vi "Begin.vi"(8 "error in":errorcluster) -> (0 "error out":errorcluster)   [LabVIEW 2017]
doc: "Called before other user functions, this VI is expected to open initial I/O refnums, load in file data, and do all program initialization. Notice that the <B>error out</B> terminal is simply used for data flow. Wiring it to other structures or subVIs ensures that this VI runs first."
uses:
  <vilib>/Rock Robotics/WPI/DriverStation/WPI_DriverStationRobotMode2.ctl
  <vilib>/Rock Robotics/WPI/Joystick/WPI_JoystickDeviceEnum.ctl
  <vilib>/Rock Robotics/WPI/Solenoid/WPI_SolenoidChannel.ctl
  <vilib>/Rock Robotics/SystemInterfaces/DIO/FPGA_DIOChannel.ctl
  Robot Global Data.vi
  <vilib>/Rock Robotics/WPI/Solenoid/WPI_SolenoidOpenSingle.vi
  <vilib>/Rock Robotics/WPI/Counter/WPI_CounterDigitalInputToDigitalSource.vi
  <vilib>/Rock Robotics/WPI/Switch/WPI_SwitchOpenLimit.vi
  <vilib>/Rock Robotics/WPI/Utilities/WPI_GetSetVariantRefNum.vi
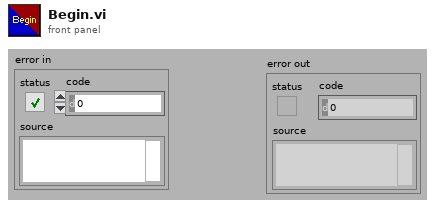
[diagram p1: front panel]
types:
  T1 = typedef "WPI_SolenoidChannel.ctl" = enum8{"Solenoid 0", "Solenoid 1", "Solenoid 2", "Solenoid 3", "Solenoid 4", "Solenoid 5", "Solenoid 6", "Solenoid 7", "Invalid"}
  T2 = typedef "FPGA_DIOChannel.ctl" = enum8{"DIO 0", "DIO 1", "DIO 2", "DIO 3", "DIO 4", "DIO 5", "DIO 6", "DIO 7", "DIO 8", "DIO 9", "DIO MXP 0", "DIO MXP 1", "DIO MXP 2", "DIO MXP 3", "DIO MXP 4", "DIO MXP 5", "DIO MXP 6", "DIO MXP 7", "DIO MXP 8", "DIO MXP 9", "DIO MXP 10", "DIO MXP 11", "DIO MXP 12", "DIO MXP 13", "DIO MXP 14", "DIO MXP 15", "SPI Port CS1", "SPI Port CS2", "SPI Port CS3", "SPI Port MISO", "SPI Port MOSI", "Invalid"}
  T3 = typedef "WPI_JoystickDeviceEnum.ctl" = enum16{"USB 0", "USB 1", "USB 2", "USB 3", "USB 4", "USB 5"}
  T4 = typedef "WPI_DriverStationRobotMode2.ctl" = enum16{"Autonomous Disabled", "Autonomous Enabled", "Teleop Disabled", "Teleop Enabled", "Disconnected", "Finish", "Test Disabled", "Test Enabled", "Emergency Stopped"}
  T5 = typedef "WPI_CompressorDevRef.ctl" = cluster{"DevStatus":errorcluster, "Pneumatics Control Module":u8}
  T6 = typedef "WPI_SwitchDevRef.ctl" = cluster{"DevStatus":errorcluster, "DIO Channel":T2, "CntIndex":T7, "Normally Closed":bool}
  T7 = typedef "FPGA_CounterCtrSystemIndex.ctl" = enum8{"Ctr 0", "Ctr 1", "Ctr 2", "Ctr 3", "Ctr 4", "Ctr 5", "Ctr 6", "Ctr 7", "Invalid"}
  T8 = typedef "WPI_DigitalInputDevRef.ctl" = cluster{"DevStatus":errorcluster, "DIO Channel":T2}
  T9 = typedef "WPI_SolenoidDevRef.ctl" = cluster{"DevStatus":errorcluster, "Pneumatics Control Module":u8, "Forward Solenoid Channel":T1, "Reverse Solenoid Channel":T1}
  T10 = typedef "FPGA_CounterEncoderSourceConvertionLVSourceType.ctl" = cluster{"DevStatus":errorcluster, "AnalogTriggerMode?":bool, "DigitalMode":cluster{"DIO Channel":T11}, "AnalogTriggerMode":cluster{"AnalogTriggerIndex":T12, "OutputType":T13}}
  T11 = typedef "FPGA_DIODigitalSourceChannel.ctl" = enum8{"DIO 0", "DIO 1", "DIO 2", "DIO 3", "DIO 4", "DIO 5", "DIO 6", "DIO 7", "DIO 8", "DIO 9", "DIO MXP 0", "DIO MXP 1", "DIO MXP 2", "DIO MXP 3", "DIO MXP 4", "DIO MXP 5", "DIO MXP 6", "DIO MXP 7", "DIO MXP 8", "DIO MXP 9", "DIO MXP 10", "DIO MXP 11", "DIO MXP 12", "DIO MXP 13", "DIO MXP 14", "DIO MXP 15", "Disabled"}
  T12 = typedef "FPGA_AnalogTriggerIndex.ctl" = enum8{"Trig 0", "Trig 1", "Trig 2", "Trig 3", "Trig 4", "Trig 5", "Trig 6", "Trig 7", "Invalid"}
  T13 = typedef "FPGA_AnalogTriggerOutType.ctl" = enum16{"InWindow", "TriggerState", "Rising", "Falling"}
  T14 = typedef "WPI_JoystickDevRef.ctl" = cluster{"Device":T3}
  T15 = typedef "WPI_EncoderDevRef.ctl" = cluster{"DevStatus":errorcluster, "EncoderIndex":T16, "CounterIndex":T7, "DistancePerCount":dbl, "Decoding Type":T17}
  T16 = typedef "FPGA_EncoderIdx.ctl" = enum8{"Enc 0", "Enc 1", "Enc 2", "Enc 3", "Enc 4", "Enc 5", "Enc 6", "Enc 7", "Invalid"}
  T17 = typedef "WPI_EncoderType.ctl" = enum16{"1x", "2x", "4x"}
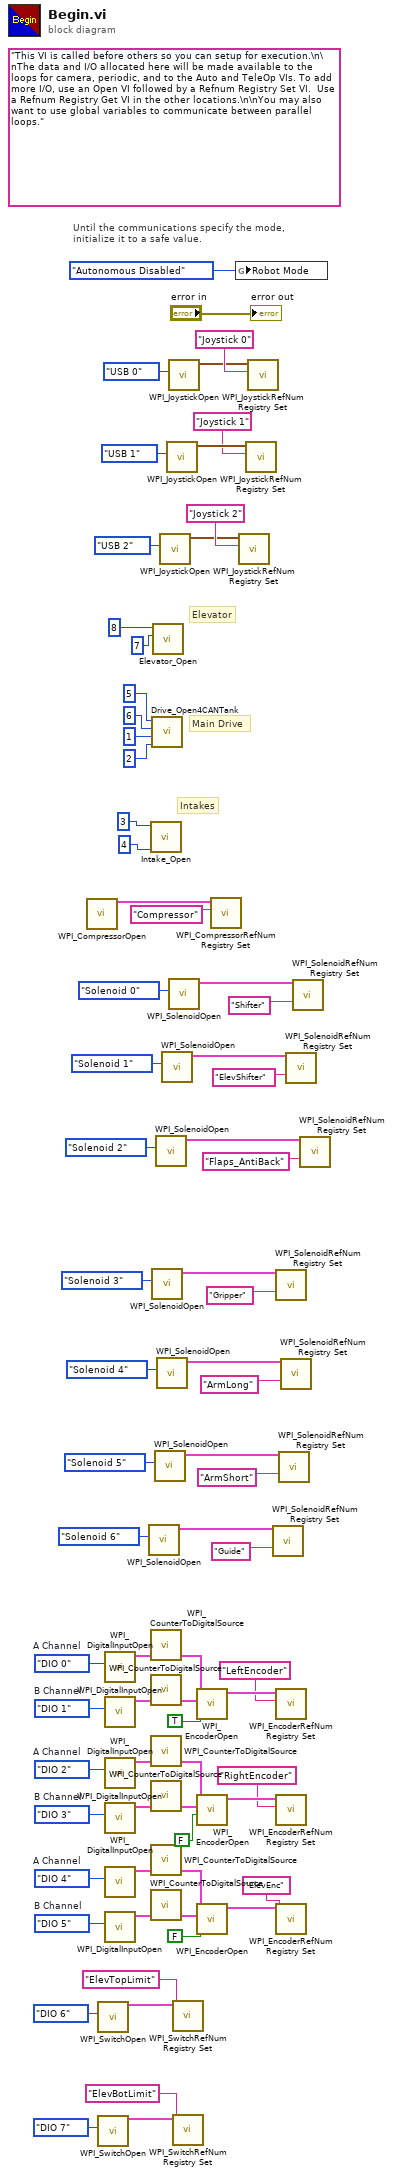
[diagram p0: block diagram]
diagram:
  w28 = FPGA_DIOChannel."DIO 5"  # B Channel
  w29 = FPGA_DIOChannel."DIO 4"  # A Channel
  w44 = FPGA_DIOChannel."DIO 3"  # B Channel
  w45 = FPGA_DIOChannel."DIO 2"  # A Channel
  w55 = FPGA_DIOChannel."DIO 1"  # B Channel
  w54 = FPGA_DIOChannel."DIO 0"  # A Channel
  (unwired) "This VI is called before others so you can setup for execution.\n\nThe data and I/O allocated here will be made available to the loops for camera, periodic, and to the Auto and TeleOp VIs. To add more I/O, use an Open VI followed by a Refnum Registry Set VI.  Use a Refnum Registry Get VI in the other locations.\n\nYou may also want to use global variables to communicate between parallel loops."
  # "Elevator"
  # "Intakes"
  # "Main Drive"
  # "Until the communications specify the mode,\ninitialize it to a safe value."
  n1 = call <vilib>:"WPI_CompressorOpen.vi"() -> ("CompressorDevRef"=w63:T5)  [unwired: 14 in, 1 out]
  n2 = call-poly <vilib>:"WPI_SwitchOpen.vi"("DIO Channel"=FPGA_DIOChannel."DIO 6") -> ("SwitchDevRef"=w15:T6)  [unwired: 9 in, 1 out]
  n3 = call-poly <vilib>:"WPI_SwitchOpen.vi"("DIO Channel"=FPGA_DIOChannel."DIO 7") -> ("SwitchDevRef"=w12:T6)  [unwired: 9 in, 1 out]
  n4 = call <vilib>:"WPI_DigitalInputOpen.vi"("DIO Channel"=w54) -> ("DigitalInputDevRef"=w51:T8)  [unwired: 1 in, 9 out]
  n5 = call <vilib>:"WPI_DigitalInputOpen.vi"("DIO Channel"=w55) -> ("DigitalInputDevRef"=w52:T8)  [unwired: 1 in, 9 out]
  n6 = call <vilib>:"WPI_DigitalInputOpen.vi"("DIO Channel"=w45) -> ("DigitalInputDevRef"=w48:T8)  [unwired: 1 in, 9 out]
  n7 = call <vilib>:"WPI_DigitalInputOpen.vi"("DIO Channel"=w44) -> ("DigitalInputDevRef"=w47:T8)  [unwired: 1 in, 9 out]
  n8 = call <vilib>:"WPI_DigitalInputOpen.vi"("DIO Channel"=w29) -> ("DigitalInputDevRef"=w32:T8)  [unwired: 1 in, 9 out]
  n9 = call <vilib>:"WPI_DigitalInputOpen.vi"("DIO Channel"=w28) -> ("DigitalInputDevRef"=w31:T8)  [unwired: 1 in, 9 out]
  n10 = call-poly <vilib>:"WPI_SolenoidOpen.vi"("Solenoid Channel"=WPI_SolenoidChannel."Solenoid 6") -> ("SolenoidDevRef"=w3:T9)  [unwired: 9 in, 1 out]
  n11 = call "Intake_Open.vi"("LeftID"=u8 3 ("MasterID"), "RightID"=u8 4 ("SlaveID")) -> ()  [unwired: 9 in]
  n12 = call-poly <vilib>:"WPI_CounterToDigitalSource.vi"("DigitalInputDevRef"=w51) -> ("Digital Source"=w50:T10)  [unwired: 6 out]
  n13 = call-poly <vilib>:"WPI_CounterToDigitalSource.vi"("DigitalInputDevRef"=w52) -> ("Digital Source"=w53:T10)  [unwired: 6 out]
  n14 = call-poly <vilib>:"WPI_CounterToDigitalSource.vi"("DigitalInputDevRef"=w48) -> ("Digital Source"=w49:T10)  [unwired: 6 out]
  n15 = call-poly <vilib>:"WPI_CounterToDigitalSource.vi"("DigitalInputDevRef"=w47) -> ("Digital Source"=w46:T10)  [unwired: 6 out]
  n16 = call-poly <vilib>:"WPI_CounterToDigitalSource.vi"("DigitalInputDevRef"=w32) -> ("Digital Source"=w33:T10)  [unwired: 6 out]
  n17 = call-poly <vilib>:"WPI_CounterToDigitalSource.vi"("DigitalInputDevRef"=w31) -> ("Digital Source"=w30:T10)  [unwired: 6 out]
  n18 = call "Drive_Open4CANTank.vi"("RightSlaveID"=u8 2, "RightMasterID"=u8 1, "LeftSlaveID"=u8 6, "LeftMasterID"=u8 5) -> ()  [unwired: 8 in]
  n19 = call-poly <vilib>:"WPI_SolenoidOpen.vi"("Solenoid Channel"=WPI_SolenoidChannel."Solenoid 3") -> ("SolenoidDevRef"=w25:T9)  [unwired: 9 in, 1 out]
  n20 = call "Elevator_Open.vi"("ElevatorSlaveID"=u8 7 ("ClimbSlave1ID"), "ElevatorMasterID"=u8 8 ("ClimbMasterID")) -> ()  [unwired: 10 in]
  n21 = call-poly <vilib>:"WPI_SolenoidOpen.vi"("Solenoid Channel"=WPI_SolenoidChannel."Solenoid 5") -> ("SolenoidDevRef"=w19:T9)  [unwired: 9 in, 1 out]
  n22 = call-poly <vilib>:"WPI_SolenoidOpen.vi"("Solenoid Channel"=WPI_SolenoidChannel."Solenoid 2") -> ("SolenoidDevRef"=w6:T9)  [unwired: 9 in, 1 out]
  n23 = call-poly <vilib>:"WPI_SolenoidOpen.vi"("Solenoid Channel"=WPI_SolenoidChannel."Solenoid 4") -> ("SolenoidDevRef"=w24:T9)  [unwired: 9 in, 1 out]
  n24 = call <vilib>:"WPI_JoystickOpen.vi"("JoystickDevice"=WPI_JoystickDeviceEnum."USB 2") -> ("JoystickDevRef"=w57:T14)  [unwired: 10 in]
  n25 = call-poly <vilib>:"WPI_SolenoidOpen.vi"("Solenoid Channel"=WPI_SolenoidChannel."Solenoid 1") -> ("SolenoidDevRef"=w7:T9)  [unwired: 9 in, 1 out]
  n26 = call <vilib>:"WPI_JoystickOpen.vi"("JoystickDevice"=WPI_JoystickDeviceEnum."USB 1") -> ("JoystickDevRef"=w65:T14)  [unwired: 10 in]
  n27 = call <vilib>:"WPI_JoystickOpen.vi"("JoystickDevice"=WPI_JoystickDeviceEnum."USB 0") -> ("JoystickDevRef"=w73:T14)  [unwired: 10 in]
  n28 = call-poly <vilib>:"WPI_SolenoidOpen.vi"("Solenoid Channel"=WPI_SolenoidChannel."Solenoid 0") -> ("SolenoidDevRef"=w61:T9)  [unwired: 9 in, 1 out]
  n29 = call <vilib>:"WPI_SwitchRefNum Registry Set.vi"("refnum name"="ElevTopLimit", "SwitchDevRef"=w15) -> ()  [unwired: 8 in, 2 out]
  n30 = call <vilib>:"WPI_SwitchRefNum Registry Set.vi"("refnum name"="ElevBotLimit", "SwitchDevRef"=w12) -> ()  [unwired: 8 in, 2 out]
  n31 = call <vilib>:"WPI_EncoderOpen.vi"("Invert Direction (False)"=TRUE, "BSource"=w53, "ASource"=w50) -> ("EncoderDevRef"=w43:T15)  [unwired: 5 in, 3 out]
  n32 = call <vilib>:"WPI_EncoderOpen.vi"("Invert Direction (False)"=FALSE, "BSource"=w46, "ASource"=w49) -> ("EncoderDevRef"=w42:T15)  [unwired: 5 in, 3 out]
  n33 = call <vilib>:"WPI_EncoderOpen.vi"("Invert Direction (False)"=FALSE, "BSource"=w30, "ASource"=w33) -> ("EncoderDevRef"=w34:T15)  [unwired: 5 in, 3 out]
  n34 = call <vilib>:"WPI_CompressorRefNum Registry Set.vi"("refnum name"="Compressor", "CompressorDevRef"=w63) -> ()  [unwired: 8 in, 2 out]
  n35 = global write "Robot Global Data.vi" "Robot Mode"(WPI_DriverStationRobotMode2."Autonomous Disabled" ("Robot Mode")) -> ()
  n36 = call <vilib>:"WPI_JoystickRefNum Registry Set.vi"("refnum name"="Joystick 2", "JoystickDevRef"=w57) -> ()  [unwired: 8 in, 2 out]
  n37 = call <vilib>:"WPI_JoystickRefNum Registry Set.vi"("refnum name"="Joystick 1", "JoystickDevRef"=w65) -> ()  [unwired: 8 in, 2 out]
  n38 = call <vilib>:"WPI_JoystickRefNum Registry Set.vi"("refnum name"="Joystick 0", "JoystickDevRef"=w73) -> ()  [unwired: 8 in, 2 out]
  n39 = call <vilib>:"WPI_SolenoidRefNum Registry Set.vi"("refnum name"="Guide", "SolenoidDevRef"=w3) -> ()  [unwired: 8 in, 2 out]
  n40 = call <vilib>:"WPI_SolenoidRefNum Registry Set.vi"("refnum name"="Gripper", "SolenoidDevRef"=w25) -> ()  [unwired: 8 in, 2 out]
  n41 = call <vilib>:"WPI_EncoderRefNum Registry Set.vi"("refnum name"="LeftEncoder", "EncoderDevRef"=w43) -> ()  [unwired: 8 in, 2 out]
  n42 = call <vilib>:"WPI_EncoderRefNum Registry Set.vi"("refnum name"="RightEncoder", "EncoderDevRef"=w42) -> ()  [unwired: 8 in, 2 out]
  n43 = call <vilib>:"WPI_EncoderRefNum Registry Set.vi"("refnum name"="ElevEnc", "EncoderDevRef"=w34) -> ()  [unwired: 8 in, 2 out]
  n44 = call <vilib>:"WPI_SolenoidRefNum Registry Set.vi"("refnum name"="ArmShort", "SolenoidDevRef"=w19) -> ()  [unwired: 8 in, 2 out]
  n45 = call <vilib>:"WPI_SolenoidRefNum Registry Set.vi"("refnum name"="ArmLong", "SolenoidDevRef"=w24) -> ()  [unwired: 8 in, 2 out]
  n46 = call <vilib>:"WPI_SolenoidRefNum Registry Set.vi"("refnum name"="ElevShifter", "SolenoidDevRef"=w7) -> ()  [unwired: 8 in, 2 out]
  n47 = call <vilib>:"WPI_SolenoidRefNum Registry Set.vi"("refnum name"="Shifter", "SolenoidDevRef"=w61) -> ()  [unwired: 8 in, 2 out]
  n48 = call <vilib>:"WPI_SolenoidRefNum Registry Set.vi"("refnum name"="Flaps_AntiBack", "SolenoidDevRef"=w6) -> ()  [unwired: 8 in, 2 out]
  "error out" <- "error in"
